vi "1820_PS_ON_duration.vi"(10 "SWITCH HEATER":bool, 11 "time stamp":timestamp format="%<%I:%M:%S %p>T") -> (3 "PS Heat on (sec)":dbl)   [LabVIEW 2016]
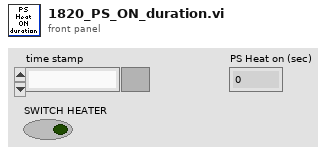
[diagram p1: front panel]
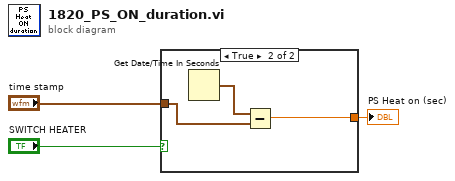
[diagram p0: block diagram]
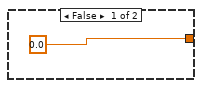
[diagram p2: hidden frame]
diagram:
  n1 = case shown="True" "SWITCH HEATER" {
    tunnel: "time stamp" -> [_ w6]
    tunnel: [0.0 ("LPF on (s)") w5] -> w1
    frame False {
    }
    frame True {
      n2 = Get Date/Time In Seconds() -> (seconds since 1Jan1904=w7:timestamp)
      n3 = Subtract(x=w7, y=w6) -> (x-y=w5:dbl)
    }
  }
  "PS Heat on (sec)" <- w1
